vi "MinerMain.vi"() -> ()   [LabVIEW 2014]
panel:
  in  "stop":bool
  out "i":i32
  out "concatenated string":string
  out "job":string="2.4"
  out "FeedBack":string="2.4"
  in  "chipID":string="1"
  in  "RIG_IDENTIFIER":string="LabVIEW"
  out "error out":errorcluster={"status"=FALSE, "code"=66, "source"=""}
  in  "UserName":string="trump"
  out "版本号":string
  in  "远程端口或服务名称":u16=6004
  in  "HostIP":string="149.91.88.18"
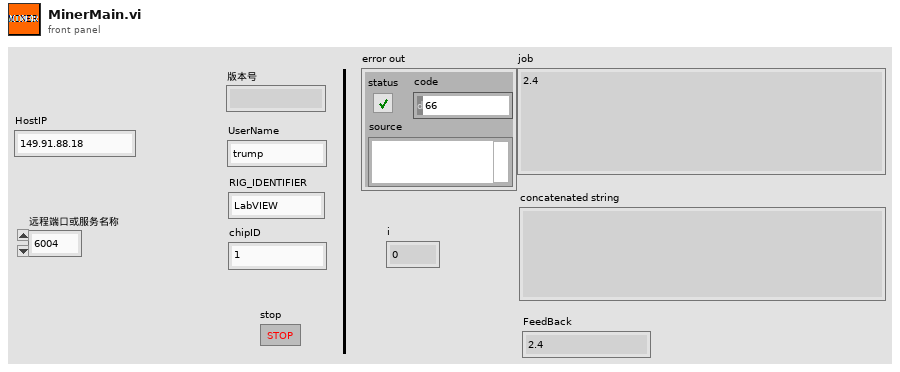
[diagram p1: front panel]
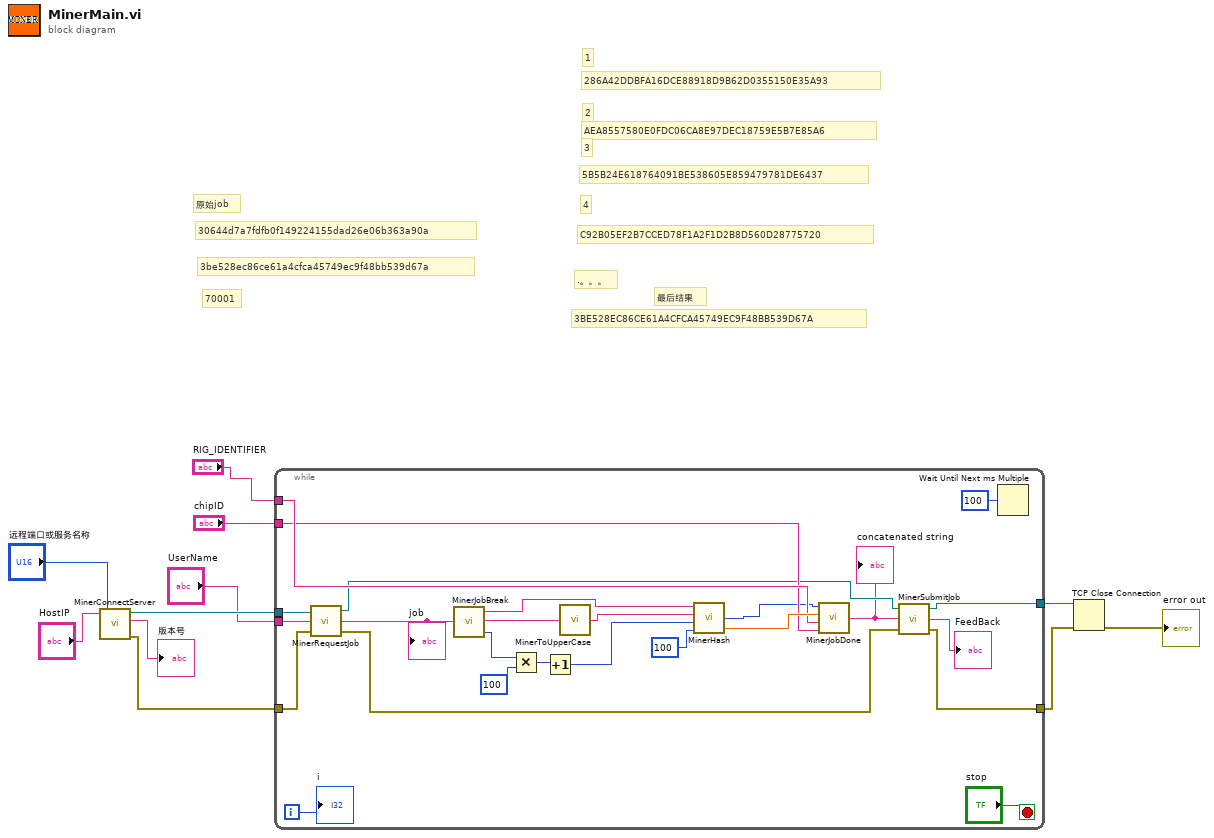
[diagram p0: block diagram]
diagram:
  # "最后结果"
  # "3BE528EC86CE61A4CFCA45749EC9F48BB539D67A"
  # ".。。。"
  # "C92B05EF2B7CCED78F1A2F1D2B8D560D28775720"
  # "4"
  # "3"
  # "5B5B24E618764091BE538605E859479781DE6437"
  # "2"
  # "AEA8557580E0FDC06CA8E97DEC18759E5B7E85A6"
  # "1"
  # "286A42DDBFA16DCE88918D9B62D0355150E35A93"
  # "原始job"
  # "70001"
  # "3be528ec86ce61a4cfca45749ec9f48bb539d67a"
  # "30644d7a7fdfb0f149224155dad26e06b363a90a"
  n1 = call "MinerConnectServer.vi"("HostIP"="HostIP", "远程端口或服务名称"="远程端口或服务名称") -> ("connection ID out"=w8:refnum<k5>, "版本号"=→"版本号":string, "错误输出 2"=w9:errorcluster)  [unwired: 1 in, 1 out]
  n2 = while {
    tunnel: w8 -> [w35]
    tunnel: "UserName" -> [w34]
    tunnel: "RIG_IDENTIFIER" -> [w22]
    tunnel: "chipID" -> [w21]
    tunnel: [w16] -> w3
    tunnel: w9 -> [w36]
    tunnel: [w18] -> w2
    i -> [w14]
    stop <- "stop" stop-if-true
    n3 = call "MinerRequestJob.vi"("error in (no error)"=w36, "UserName"=w34, "connection ID"=w35) -> ("error out"=w19:errorcluster, "job"=w33:string, "connection ID out"=w20:refnum<k5>)
    "job" <- w33
    n4 = call "MinerJobBreak.vi"("JOB"=w33) -> ("difficulty"=w32:i32, "expected"=w29:string, "last_block"=w27:string)  [unwired: 2 in]
    n5 = Multiply(x=w32, y=100) -> (x*y=w30:i32)
    n6 = Increment(x=w30) -> (x+1=w26:i32)
    n7 = call "MinerToUpperCase.vi"("expected"=w29) -> ("UpperExpected"=w28:string)
    n8 = call "MinerHash.vi"("TimeDelay"=u32 100, "difficulty"=w26, "expected"=w28, "last_block"=w27) -> ("elapsed_time_s"=w24:dbl, "duco_numeric_result"=w13:i32)  [unwired: 1 out]
    n9 = call "MinerJobDone.vi"("chipID"=w21, "RIG_IDENTIFIER"=w22, "hashrate"=w24, "duco_numeric_result"=w13) -> ("concatenated string"=w17:string)
    "concatenated string" <- w17
    n10 = call "MinerSubmitJob.vi"("error in (no error)"=w19, "JobDoneString"=w17, "connection ID"=w20) -> ("error out"=w18:errorcluster, "FeedBack"=→"FeedBack":string, "connection ID out"=w16:refnum<k5>)
    n11 = Wait Until Next ms Multiple(millisecond multiple=u32 100) -> ()  [unwired: 1 out]
    "i" <- w14
  }
  n12 = TCP Close Connection(connection ID=w3, error in (no error)=w2) -> (error out=→"error out":errorcluster)  [unwired: 1 in, 1 out]
